vi "WHH Fit.vi"() -> ()   [LabVIEW 2021]
uses:
  WHH Formula Data.ctl
  <vilib>/gmath/zero.llb/Newton Raphson Zero Finder (VI).vi
  <vilib>/gmath/NI_Gmath.lvlib
panel:
  in  "lambda_SO":dbl
  in  "alpha_Maki":dbl
  out "Array - Numeric":dbl[](array[numeric])
  out "XY Graph":cluster{dbl[], "Steps":dbl[]}(graph)
  in  "Number of steps":i32=100
  in  "End":dbl=0.9999
  in  "Start":dbl=0.0001
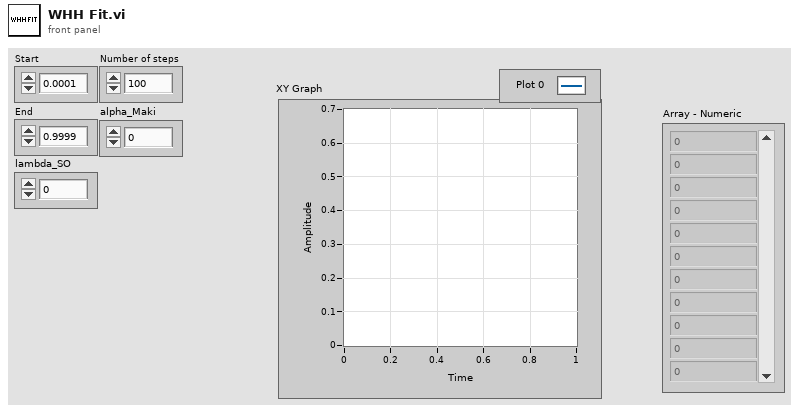
[diagram p1: front panel]
types:
  T1 = typedef "WHH Formula Data.ctl" = cluster{"t":dbl, "alpha_Maki":dbl, "lambda_SO":dbl}
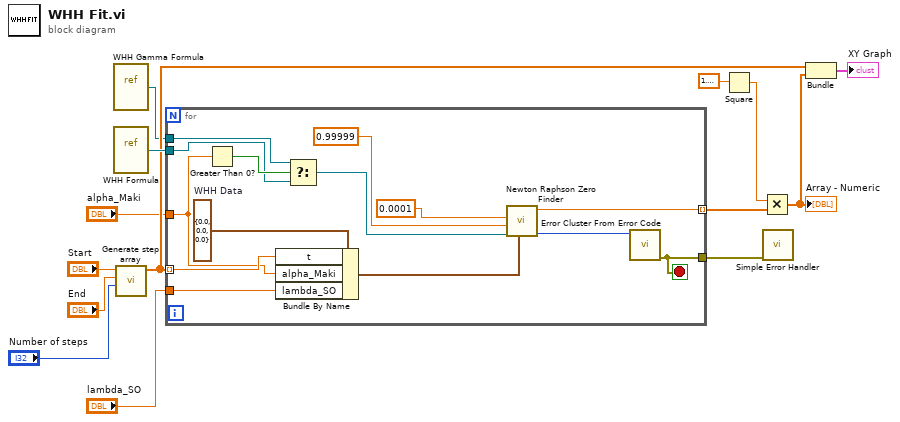
[diagram p0: block diagram]
diagram:
  n1 = vi-ref "WHH Gamma Formula.vi"() -> (w1:refnum<vi>)
  n2 = vi-ref "WHH Formula.vi"() -> (w9:refnum<vi>)
  n3 = call "Generate step array.vi"("Number of steps"="Number of steps", "End"="End", "Start"="Start") -> ("Steps"=w8:dbl[])  [unwired: 8 in]
  n4 = for {
    tunnel: w9 -> [w18]
    tunnel: w8 -> [w28] mode=indexing
    tunnel: [w25] -> w5 mode=indexing
    tunnel: [w23] -> w10
    tunnel: "alpha_Maki" -> [w21]
    tunnel: "lambda_SO" -> [w22]
    tunnel: w1 -> [w19]
    stop <- w23 stop-if-true
    w27 = T1 {"t"=0.0, "alpha_Maki"=0.0, "lambda_SO"=0.0}  # WHH Data
    n5 = Greater Than 0?(x=w21) -> (x > 0?=w20:bool)
    n6 = Bundle By Name(cluster=w27, "t"=w28, "alpha_Maki"=w21, "lambda_SO"=w22) -> (w26:T1)
    n7 = Select(t=w19, s=w20, f=w18) -> (s? t:f=w17:refnum<vi>)
    n8 = call-poly <vilib>:"Newton Raphson Zero Finder.vi"("data"=w26, "f(x)"=w17, "end"=0.99999, "start"=0.0001) -> ("error"=w24:i32, "zero"=w25:dbl)  [unwired: 4 in, 2 out]
    n9 = call <vilib>:"Error Cluster From Error Code.vi"("error code (0)"=w24) -> ("error out"=w23:errorcluster)  [unwired: 8 in]
  }
  n10 = Square(x=1.5707963267948966) -> (x^2=w6:dbl)
  n11 = Multiply(x=w6, y=w5) -> (x*y=w4:dbl[])
  "Array - Numeric" <- w4
  n12 = call <vilib>:"Simple Error Handler.vi"("error in (no error)"=w10) -> ()  [unwired: 4 in, 5 out]
  n13 = Bundle("Steps"=w8, w4) -> (→"XY Graph":cluster{"Steps":dbl[], dbl[]})  [unwired: 1 in]
